vi "SUBVI_get_pixel_sensor_offset.vi"(4 "vertical binning":dbl, 5 "y dim":dbl, 6 "horizontal binning":dbl, 7 "x dim":dbl, 9 "max height":dbl, 11 "max width":dbl) -> (1 "y offset":dbl, 3 "x offset":dbl)   [LabVIEW 2020]
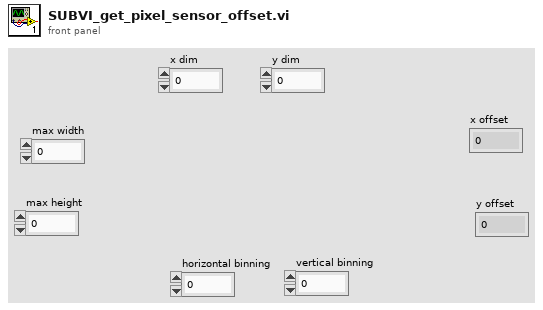
[diagram p1: front panel]
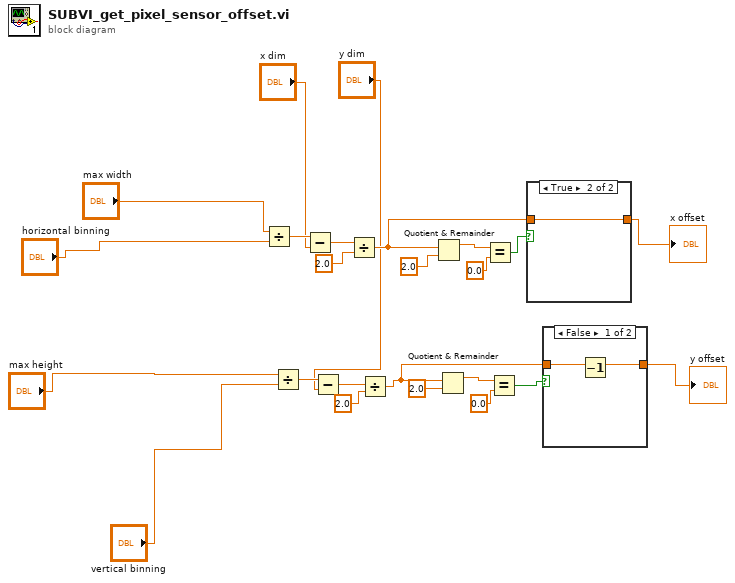
[diagram p0: block diagram]
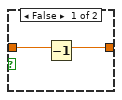
[diagram p3: hidden frame]
diagram:
  n1 = Divide(x="max width", y="horizontal binning") -> (x/y=w20:dbl)
  n2 = Divide(x="max height", y="vertical binning") -> (x/y=w21:dbl)
  n3 = Subtract(x=w20, y="x dim") -> (x-y=w22:dbl)
  n4 = Subtract(x=w21, y="y dim") -> (x-y=w23:dbl)
  n5 = Divide(x=w22, y=2.0) -> (x/y=w5:dbl)
  n6 = Divide(x=w23, y=2.0) -> (x/y=w6:dbl)
  n7 = Quotient & Remainder(x=w5, y=2.0) -> (x-y*floor(x/y)=w13:dbl)  [unwired: 1 out]
  n8 = Quotient & Remainder(x=w6, y=2.0) -> (x-y*floor(x/y)=w7:dbl)  [unwired: 1 out]
  n9 = Equal?(x=w13, y=0.0) -> (x = y?=w14:bool)
  n10 = Equal?(x=w7, y=0.0) -> (x = y?=w8:bool)
  n11 = case shown="True" w14 {
    tunnel: w5 -> [w26 w27]
    tunnel: [w25 w27] -> w12
    frame False {
      n12 = Decrement(x=w26) -> (x-1=w25:dbl)
    }
    frame True {
    }
  }
  "x offset" <- w12
  n13 = case shown="False" w8 {
    tunnel: w6 -> [w29 w30]
    tunnel: [w28 w30] -> w9
    frame False {
      n14 = Decrement(x=w29) -> (x-1=w28:dbl)
    }
    frame True {
    }
  }
  "y offset" <- w9
